vi "toolbox_error_handler.vi"(6 "name of caller in (you)":string, 8 "error in (no error)":errorcluster, 9 "additional info":string, 10 "code (0 = no error)":i32) -> (0 "error out":errorcluster, 1 "error in self?":bool)   [LabVIEW 2015]
uses:
  polys/poly_global_eco_plus.vi
  cores/core_global_ECO.vi
  cores/core_is_code_plus_eco.vi
  polys/poly_global_eco_minus.vi
  <vilib>/Utility/error.llb/Error Code Database.vi
panel:
  # "ECO = Error Code Offset"
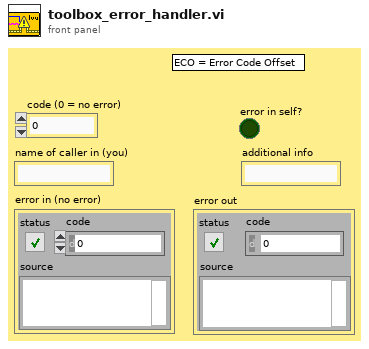
[diagram p1: front panel]
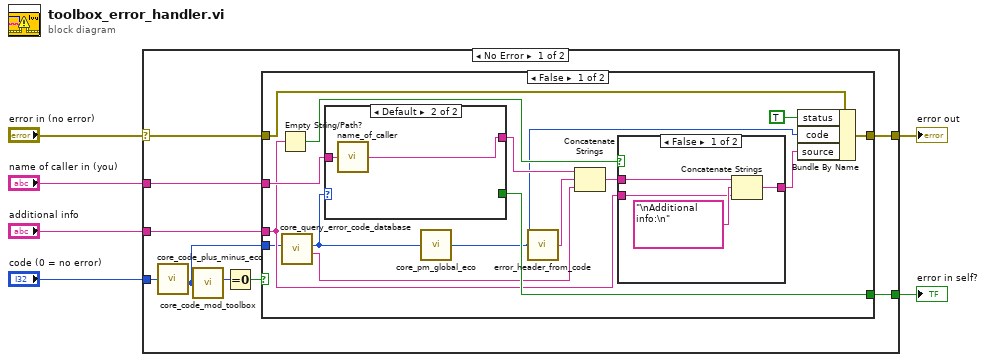
[diagram p0: block diagram]
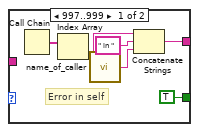
[diagram p3: hidden frame]
diagram:
  n1 = case shown="No Error" "error in (no error)" {
    selector: "error in (no error)" -> [w9 w45]
    tunnel: "name of caller in (you)" -> [w15 _]
    tunnel: "code (0 = no error)" -> [w10 _]
    tunnel: [w13 _] -> w4
    tunnel: [w12 w45] -> w2
    tunnel: "additional info" -> [w11 _]
    frame No Error {
      n2 = call "core_code_plus_minus_eco.vi"("code in"=w10) -> ("code w/out ECO"=w8:i32)  [unwired: 8 in, 1 out]
      n3 = call "core_code_mod_toolbox.vi"("error code"=w8) -> ("local code"=w7:i32)  [unwired: 8 in, 1 out]
      n4 = Equal To 0?(x=w7) -> (x = 0?=w14:bool)
      n5 = case shown="False" w14 {
        tunnel: w9 -> [w30 w44]
        tunnel: [w29 w44] -> w12
        tunnel: w8 -> [w18 _]
        tunnel: w15 -> [w28 _]
        tunnel: [w25 _] -> w13
        tunnel: w11 -> [w21 _]
        frame False {
          n6 = Empty String/Path?(string/path=w21) -> (empty?=w24:bool)
          n7 = call "core_query_error_code_database.vi"("code in"=w18) -> ("code description"=w16:string, "code out"=w17:i32)  [unwired: 9 in]
          n8 = case shown="Default" w17 {
            tunnel: w28 -> [_ w43]
            tunnel: [w37 w42] -> w27
            tunnel: [TRUE _] -> w25
            frame 997..999 {
              # "Error in self"
              # "Error in this vi"
              n9 = Call Chain() -> (call chain=w41:string[])
              n10 = Index Array(array=w41) -> (element=w40:string)  [unwired: 1 in]
              n11 = call "name_of_caller.vi"() -> ("name of caller out"=w38:string)  [unwired: 4 in]
              n12 = Concatenate Strings(w40, " in " ("string"), w38) -> (w37:string)
            }
            frame Default {
              n13 = call "name_of_caller.vi"("name of caller in"=w43) -> ("name of caller out"=w42:string)  [unwired: 3 in]
            }
          }
          n14 = call-poly "core_pm_global_eco.vi"("code (w/out ECO)"=w17) -> ("code (+ ECO)"=w20:i32)  [unwired: 4 in]
          n15 = call "error_header_from_code.vi"("error code"=w20) -> ("error header"=w19:string)  [unwired: 4 in]
          n16 = Concatenate Strings(w27, w19, w16) -> (w23:string)
          n17 = case shown="False" w24 {
            tunnel: w23 -> [w34 w35]
            tunnel: [w31 w35] -> w22
            tunnel: w21 -> [w32 _]
            frame False {
              n18 = Concatenate Strings(w34, "\nAdditional info:\n" ("string"), w32) -> (w31:string)
            }
            frame True {
            }
          }
          n19 = Bundle By Name(cluster=w30, "status"=TRUE, "code"=w20, "source"=w22) -> (w29:errorcluster)
        }
        frame True {
        }
      }
    }
    frame Error {
    }
  }
  "error out" <- w2
  "error in self?" <- w4
